vi "Delta Time.vi"(11 "Relative Seconds In":dbl format="%_19f") -> (2 "Delta Seconds":dbl format="%.3p", 3 "Relative Seconds Out":dbl format="%_19f")   [LabVIEW 2020, in "Utility.lvlib"]
uses:
  Utility.lvlib
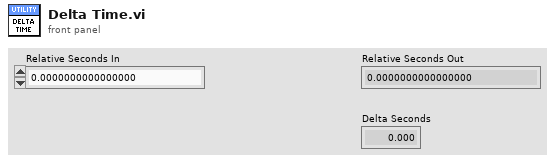
[diagram p1: front panel]
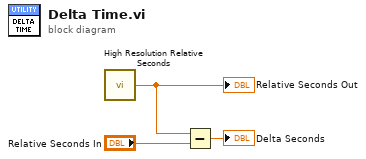
[diagram p0: block diagram]
diagram:
  n1 = call <vilib>:"High Resolution Relative Seconds.vi"() -> ("relative seconds"=w1:dbl)
  "Relative Seconds Out" <- w1
  n2 = Subtract(x=w1, y="Relative Seconds In") -> (x-y=→"Delta Seconds":dbl)
